vi "ROSmsg_isStd.vi"(10 "Data Type":string) -> (2 "Is std_msgs?":bool)   [LabVIEW 2016]
doc: "Checks a data type to see if it's a standard message"
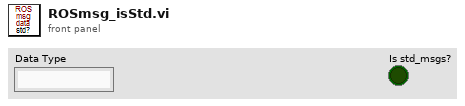
[diagram p1: front panel]
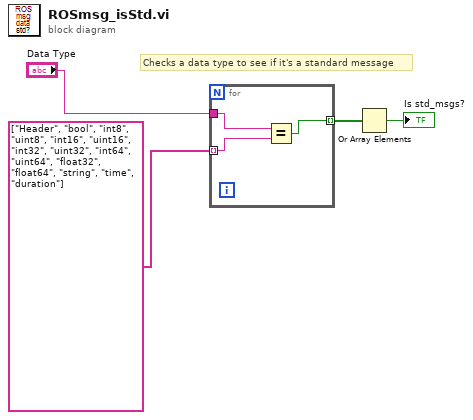
[diagram p0: block diagram]
diagram:
  # "Checks a data type to see if it's a standard message"
  n1 = for {
    tunnel: "Data Type" -> [w7]
    tunnel: string[] ["Header", "bool", "int8", "uint8", "int16", "uint16", "int32", "uint32", "int64", "uint64", "float32", "float64", "string", "time", "duration"] -> [w6] mode=indexing
    tunnel: [w5] -> w2 mode=indexing
    n2 = Equal?(x=w7, y=w6) -> (x = y?=w5:bool)
  }
  n3 = Or Array Elements(Boolean array=w2) -> (logical OR=→"Is std_msgs?":bool)
